vi "ROI entry-All or Visible.vi"(11 "Function":T1) -> (2 "Offset ALL":bool, 3 "Motor Z":dbl)   [LabVIEW 2017]
uses:
  Typedefs/ROI management FG states.ctl
  Globals/gl_ROI Entry UI globals.vi
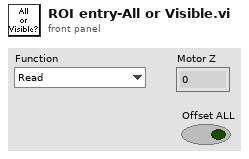
[diagram p1: front panel]
types:
  T1 = typedef "ROI management FG states.ctl" = enum16{"Read", "Write", "Clear Last", "Clear All", "Update ROIs time", "Reload last ROI set", "Offset all ROI", "Offset visible ROI"}
  T2 = typedef "ROI entry screen ctrl refs cluster.ctl" = cluster{"Done button":refnum<vi>, "Imaging button":refnum<vi>, "Acquisition button":refnum<vi>, "POI dwell time (us)":refnum<vi>, "Scan dwell time per pixel (us)":refnum<vi>, "# of planes":refnum<vi>, "Zoom Ctrl":refnum<vi>, "Equal size":refnum<vi>, "Channel":refnum<vi>, "Image Display":refnum<vi>, "Z-Plane Selector":refnum<vi>, "Number of lines left":refnum<vi>, "Z-stack folder path":refnum<vi>, "POI Density":refnum<vi>, "Arb Plane Entry":refnum<vi>, "Whole plane":refnum<vi>, "Clear Last":refnum<vi>, "Clear All":refnum<vi>, "Trial Length (sec)":refnum<vi>, "Palette Type":refnum<vi>, "Intensity slider":refnum<vi>, "# POI":refnum<vi>, "Max Z Proj":refnum<vi>, "Zplane ind":refnum<vi>, "Wavelength (nm)":refnum<vi>, "Number of Trials":refnum<vi>, "Funct stim.trig.enable":refnum<vi>, "Funct stim.trig.delay (s)":refnum<vi>, "Line Mode":refnum<vi>, "Step size (µm)":refnum<vi>, "ROI move mode":refnum<vi>, "Cool-down time (s)":refnum<vi>, "Enable cool-down time":refnum<vi>, "Motor Z ind. (um)":refnum<vi>, "AOL Z ind. (um)":refnum<vi>, "Load Reference Image":refnum<vi>}
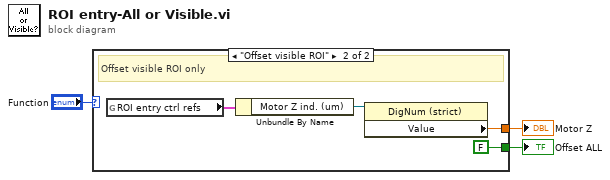
[diagram p0: block diagram]
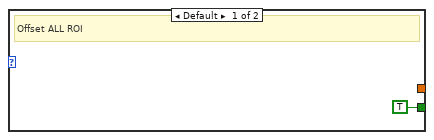
[diagram p2: hidden frame]
diagram:
  n1 = case shown="\"Offset visible ROI\"" "Function" {
    tunnel: [_ w6] -> w2
    tunnel: [TRUE FALSE] -> w1
    frame Default {
      # "Offset ALL ROI"
    }
    frame "Offset visible ROI" {
      # "Offset visible ROI only"
      n2 = global read "gl_ROI Entry UI globals.vi" "ROI entry ctrl refs"() -> (w8:T2)
      n3 = Unbundle By Name(w8) -> ("Motor Z ind. (um)"=w7:refnum<vi>)
      n4 = property class="DigNum (strict)"(reference=w7) -> ("Value"=w6:dbl)  [unwired: 1 in, 2 out]
    }
  }
  "Motor Z" <- w2
  "Offset ALL" <- w1
